vi "UHR-Fleezers Control (host) - 10.5.vi"() -> ()   [LabVIEW 2011] (continued)
          }
          frame #4 {
            n513 = property on="Trap Pos. FB ON" class="Bool (strict)"("Val(Sgnl)"=TRUE ("Value (Signaling)")) -> ()  [unwired: 2 in, 2 out]
            n514 = Wait (ms)(milliseconds to wait=u32 250) -> ()  [unwired: 1 out]
          }
          frame #5 {
            n515 = case shown="False" "Trap Trig Fl." {
              frame False {
                n516 = case shown="True" "Green ON after FB ON?" {
                  selector: "Green ON after FB ON?" -> [_ w823]
                  frame False {
                  }
                  frame True {
                    n517 = property on="Green Laser ON/Interlacing" class="Bool (strict)"("Val(Sgnl)"=w823) -> ()  [unwired: 2 in, 2 out]
                  }
                }
              }
              frame True {
              }
            }
            n518 = case shown="True" "Remove Action Offset" {
              tunnel: TRUE ("Value (Signaling)") -> [w820 w821]
              frame False {
                n519 = property on="Remove Unwinding Offset" class="Bool (strict)"("Val(Sgnl)"=w820) -> ()  [unwired: 2 in, 2 out]
              }
              frame True {
                n520 = property on="Remove Action Offset" class="Bool (strict)"("Val(Sgnl)"=w821) -> ()  [unwired: 2 in, 2 out]
              }
            }
            n521 = Wait (ms)(milliseconds to wait=u32 250) -> ()  [unwired: 1 out]
          }
          frame #6 {
            n522 = property on="Start Saving" class="Bool (strict)"("Val(Sgnl)"=TRUE ("Value (Signaling)")) -> ()  [unwired: 2 in, 2 out]
            n523 = Wait (ms)(milliseconds to wait=u32 5000) -> ()  [unwired: 1 out]
          }
          frame #7 {
            n524 = property on="Rem fb disp offset" class="Bool (strict)"("Val(Sgnl)"=TRUE ("Value (Signaling)")) -> ()  [unwired: 2 in, 2 out]
            n525 = Wait (ms)(milliseconds to wait=u32 100) -> ()  [unwired: 1 out]
          }
          frame #8 {
            n526 = case shown="True" w830 {
              frame False {
              }
              frame True {
                n527 = local write "Trap Trig. Fl."(TRUE ("Value (Signaling)")) -> ()
              }
            }
          }
          frame #9 {
            n528 = case shown="True" "Start dipping after?" {
              frame False {
              }
              frame True {
                n529 = property on="Dip for Protein" class="Bool (strict)"("Val(Sgnl)"=TRUE ("Value (Signaling)")) -> ()  [unwired: 2 in, 2 out]
                n530 = local write "Scripts"(T2."Dipping" ("Scripts")) -> ()
              }
            }
          }
        }
      }
      event "Fixed Traps Data\nScript": Value Change {
        n531 = event-data() -> ()  [unwired: 1 in, 5 out]
        n532 = flat-sequence {
          frame #0 {
            n533 = case shown="True" "Green ON" {
              frame False {
              }
              frame True {
                n534 = property on="Green Laser ON/Interlacing" class="Bool (strict)"("Val(Sgnl)"=TRUE) -> ()  [unwired: 2 in, 2 out]
              }
            }
            n535 = local write "Offset (nm)"(0.0 ("Offset (nm)")) -> ()
            n536 = property on="Sample Channel\nFlow" class="Bool (strict)"("Val(Sgnl)"=FALSE ("Value (Signaling)")) -> ()  [unwired: 2 in, 2 out]
            n537 = property on="Trap Delta (MHz)" class="DigNum (strict)"("Val(Sgnl)"="Fixed Traps Trap Delta (MHz)") -> ()  [unwired: 2 in, 2 out]
          }
          frame #1 {
            n538 = Wait (ms)(milliseconds to wait=u32 1000) -> ()  [unwired: 1 out]
          }
          frame #2 {
            n539 = local write "Start Saving"(TRUE ("Start Saving")) -> ()
          }
          frame #3 {
            n540 = local read "Bead Sep. Int. Time (s)"() -> (w842:dbl)
            n541 = Multiply(x=w842, y=1000.0) -> (x*y=w844:dbl)
            n542 = Wait (ms)(milliseconds to wait=w844) -> ()  [unwired: 1 out]
          }
          frame #4 {
            n543 = property on="Remove Offset" class="Bool (strict)"("Val(Sgnl)"=TRUE ("Value (Signaling)")) -> ()  [unwired: 2 in, 2 out]
          }
          frame #5 {
            n544 = property on="Dip for Protein" class="Bool (strict)"("Val(Sgnl)"="Start dipping after?") -> ()  [unwired: 2 in, 2 out]
          }
        }
      }
      event "Got DNA bead": Value Change {
        n545 = event-data() -> ()  [unwired: 1 in, 5 out]
        n546 = flat-sequence {
          frame #0 {
            n547 = local read "Daq spot flow on"() -> (w848:bool)
            n548 = case shown="True" w848 {
              frame False {
              }
              frame True {
                n549 = property on="Sample Channel\nFlow" class="Bool (strict)"("Val(Sgnl)"=TRUE ("Value (Signaling)")) -> ()  [unwired: 2 in, 2 out]
              }
            }
          }
          frame #1 {
            n550 = property on="Cal/Data Acq. Spot" class="Bool (strict)"("Val(Sgnl)"=TRUE ("Value (Signaling)")) -> ()  [unwired: 2 in, 2 out]
            n551 = property on="Inject Pump 1" class="Bool (strict)"("Val(Sgnl)"=FALSE ("Value (Signaling)")) -> ()  [unwired: 2 in, 2 out]
          }
        }
      }
      event "Take Stepping Data": Value Change {
        n552 = event-data() -> ()  [unwired: 1 in, 5 out]
        n553 = local read "Save ave N"() -> (w860:dbl)
        n554 = flat-sequence {
          tunnel: w860 -> [w862]
          tunnel: [w862] -> w855
          tunnel: [w864] -> w856
          tunnel: w855 -> [w864]
          tunnel: [w866] -> w857
          tunnel: w856 -> [w866]
          tunnel: [w869] -> w858
          tunnel: w857 -> [w869]
          tunnel: [w871] -> w859
          tunnel: w858 -> [w871]
          tunnel: [w873] -> w853
          tunnel: w859 -> [w873]
          tunnel: w853 -> [w876]
          tunnel: [w876] -> w852
          tunnel: w852 -> [w877]
          tunnel: [w877] -> w854
          tunnel: w854 -> [w883]
          frame #0 {
            n555 = property on="Save ave N" class="DigNum (strict)"("Val(Sgnl)"="Save ave factor") -> ()  [unwired: 2 in, 2 out]
          }
          frame #1 {
            n556 = Wait (ms)(milliseconds to wait=u32 100) -> ()  [unwired: 1 out]
          }
          frame #2 {
            n557 = local read "Offset 2 Start (MHz)"() -> (w868:dbl)
            n558 = property on="Saved AOD Raster Scan Parameter Sets" class="Arr (strict)"("Index Values"=u32[] [2]) -> ()  [unwired: 2 in, 2 out]
            n559 = property on="Trap Delta (MHz)" class="DigNum (strict)"("Val(Sgnl)"=w868) -> ()  [unwired: 2 in, 2 out]
          }
          frame #3 {
            n560 = property on="Load parameters" class="Bool (strict)"("Val(Sgnl)"=TRUE ("Value (Signaling)")) -> ()  [unwired: 2 in, 2 out]
          }
          frame #4 {
            n561 = Wait (ms)(milliseconds to wait=u32 100) -> ()  [unwired: 1 out]
          }
          frame #5 {
            n562 = property on="Trap Raster Scan" class="Bool (strict)"("Val(Sgnl)"=TRUE ("Value (Signaling)")) -> ()  [unwired: 2 in, 2 out]
          }
          frame #6 {
            n563 = Wait (ms)(milliseconds to wait=u32 1000) -> ()  [unwired: 1 out]
          }
          frame #7 {
            n564 = while {
              stop <- w880 stop-if-true
              n565 = local read "Raster Scanning..."() -> (w882:bool)
              n566 = local read "Saving..."() -> (w881:bool)
              n567 = Not(x=w881) -> (.not. x?=w878:bool)
              n568 = Not(x=w882) -> (.not. x?=w879:bool)
              n569 = And(x=w879, y=w878) -> (x .and. y?=w880:bool)
            }
          }
          frame #8 {
            n570 = property on="Save ave N" class="DigNum (strict)"("Val(Sgnl)"=w883) -> ()  [unwired: 2 in, 2 out]
          }
        }
      }
      event "Step Size (nm)": Value Change {
        n571 = event-data() -> ()  [unwired: 1 in, 5 out]
        n572 = flat-sequence {
          frame #0 {
            n573 = property on="Saved AOD Raster Scan Parameter Sets" class="Arr (strict)"("Index Values"=u32[] [1]) -> ()  [unwired: 2 in, 2 out]
          }
          frame #1 {
            n574 = Multiply(x="N Steps", y="Step Size (nm)") -> (x*y=w885:dbl)
            n575 = property on="Scan Speed AOD (nm/s) 2" class="DigNum (strict)"("Value"="Step Size (nm)") -> ()  [unwired: 2 in, 2 out]
            n576 = property on="Step Size AOD (nm) 2" class="DigNum (strict)"("Value"="Step Size (nm)") -> ()  [unwired: 2 in, 2 out]
            n577 = property on="Scan Range AOD (nm) 2" class="DigNum (strict)"("Value"=w885) -> ()  [unwired: 2 in, 2 out]
          }
        }
      }
      event "Take Detection Laser\nImage": Value Change {
        n578 = event-data() -> ()  [unwired: 1 in, 5 out]
        n579 = flat-sequence {
          tunnel: [w913] -> w903
          tunnel: [w912] -> w896
          tunnel: [w911] -> w888
          tunnel: [w916] -> w904
          tunnel: w903 -> [w916]
          tunnel: [w915] -> w897
          tunnel: w896 -> [w915]
          tunnel: [w914] -> w889
          tunnel: w888 -> [w914]
          tunnel: [w920] -> w905
          tunnel: w904 -> [w920]
          tunnel: [w919] -> w898
          tunnel: w897 -> [w919]
          tunnel: [w918] -> w890
          tunnel: w889 -> [w918]
          tunnel: [w926] -> w906
          tunnel: w905 -> [w926]
          tunnel: [w925] -> w899
          tunnel: w898 -> [w925]
          tunnel: [w924] -> w891
          tunnel: w890 -> [w924]
          tunnel: [w930] -> w907
          tunnel: w906 -> [w930]
          tunnel: [w929] -> w900
          tunnel: w899 -> [w929]
          tunnel: [w928] -> w892
          tunnel: w891 -> [w928]
          tunnel: [w934] -> w908
          tunnel: w907 -> [w934]
          tunnel: [w933] -> w901
          tunnel: w900 -> [w933]
          tunnel: [w932] -> w893
          tunnel: w892 -> [w932]
          tunnel: [w938] -> w909
          tunnel: w908 -> [w938]
          tunnel: [w937] -> w902
          tunnel: w901 -> [w937]
          tunnel: [w936] -> w894
          tunnel: w893 -> [w936]
          tunnel: w909 -> [w944]
          tunnel: w902 -> [w943]
          tunnel: [w941] -> w895
          tunnel: w894 -> [w941]
          tunnel: w895 -> [w945]
          frame #0 {
            n580 = local read "Green Laser ON/Interlacing"() -> (w913:bool)
            n581 = local read "Green laser mode"() -> (w912:enum32{"Laser ON", "Laser OFF", "Interlace"})
            n582 = local read "Green FB On/Off"() -> (w911:bool)
          }
          frame #1 {
            n583 = property on="Green FB On/Off" class="Bool (strict)"("Val(Sgnl)"=FALSE ("Value (Signaling)")) -> ()  [unwired: 2 in, 2 out]
          }
          frame #2 {
            n584 = property on="Green Laser ON/Interlacing" class="Bool (strict)"("Val(Sgnl)"=TRUE ("Value (Signaling)")) -> ()  [unwired: 2 in, 2 out]
            n585 = property on="Flip Green Filter" class="Bool (strict)"("Val(Sgnl)"=TRUE ("Value (Signaling)")) -> ()  [unwired: 2 in, 2 out]
            n586 = property on="Green laser mode" class="RadioBtnsControl (strict)"("Val(Sgnl)"=enum32{"Laser ON", "Laser OFF", "Interlace"}."Laser ON" ("Value (Signaling)")) -> ()  [unwired: 2 in, 2 out]
          }
          frame #3 {
            n587 = Wait (ms)(milliseconds to wait=u32 500) -> ()  [unwired: 1 out]
          }
          frame #4 {
            n588 = property on="Confocal Image" class="Bool (strict)"("Val(Sgnl)"=TRUE ("Value (Signaling)")) -> ()  [unwired: 2 in, 2 out]
          }
          frame #5 {
            n589 = Wait (ms)(milliseconds to wait=u32 2000) -> ()  [unwired: 1 out]
          }
          frame #6 {
            n590 = while {
              stop <- w939 stop-if-true
              n591 = local read "Saving..."() -> (w940:bool)
              n592 = Not(x=w940) -> (.not. x?=w939:bool)
            }
          }
          frame #7 {
            n593 = property on="Flip Green Filter" class="Bool (strict)"("Val(Sgnl)"=TRUE ("Value (Signaling)")) -> ()  [unwired: 2 in, 2 out]
            n594 = property on="Green Laser ON/Interlacing" class="Bool (strict)"("Val(Sgnl)"=w944) -> ()  [unwired: 2 in, 2 out]
            n595 = property on="Green laser mode" class="RadioBtnsControl (strict)"("Val(Sgnl)"=w943) -> ()  [unwired: 2 in, 2 out]
          }
          frame #8 {
            n596 = property on="Green FB On/Off" class="Bool (strict)"("Val(Sgnl)"=w945) -> ()  [unwired: 2 in, 2 out]
          }
        }
      }
      event "Stop All": Value Change {
        n597 = event-data() -> ()  [unwired: 1 in, 5 out]
        n598 = local read "Stop All"() -> (w946:bool)
      }
    }
    n599 = node-c288() -> ()  [unwired: 1 in, 1 out]
  }
  n600 = node-c288(2 ("Processor")) -> (w82:T21)  [unwired: 3 out]
  n601 = timed-loop "Control parameters (event loop)" {
    tunnel: w40 -> [w951]
    shift-right: [w950] -> _
    shift-left: errorcluster {"status"=FALSE, "code"=0, "source"=""} ("error out") -> [w949]
    tunnel: [w948] -> _
    timing: w82 -> [_]
    timing-out: [_] -> w81
    tunnel: w54 -> [w947]
    stop <- w948 stop-if-true
    n602 = node-c288() -> ()  [unwired: 2 out]
    n603 = event shown="[44] \"Sample Channel\nFlow\": Value Change" {
      selector: _ -> [_ _ _ _ _ _ _ _ _ _ _ _ _ _ _ _ _ _ _ _ _ _ _ _ _ _ _ _ _ _ _ _ _ _ _ _ _ _ _ _ _ _ _ _ _ _ _ _ _ _ _ _ _ _ _ _ _ _ _ _ _ _ _]
      dyn-events: _ -> [_ _ _ _ _ _ _ _ _ _ _ _ _ _ _ _ _ _ _ _ _ _ _ _ _ _ _ _ _ _ _ _ _ _ _ _ _ _ _ _ _ _ _ _ _ _ _ _ _ _ _ _ _ _ _ _ _ _ _ _ _ _ _]
      timeout: _ -> [_ _ _ _ _ _ _ _ _ _ _ _ _ _ _ _ _ _ _ _ _ _ _ _ _ _ _ _ _ _ _ _ _ _ _ _ _ _ _ _ _ _ _ _ _ _ _ _ _ _ _ _ _ _ _ _ _ _ _ _ _ _ _]
      tunnel: w951 -> [w989 _ _ _ w1027 _ w1049 _ _ _ _ w1115 _ _ w1158 w1164 w1169 w1175 w1211 w1229 w1236 w1247 w1251 w1262 w1273 w1284 w1295 w1306 w1317 w1344 w1438 w1445 w1483 _ w1518 w1522 w1533 w1537 w1541 _ w1549 _ _ _ _ _ _ _ w1720 _ w1737 _ w1744 w1762 _ w1769 w1777 w1792 w1803 w1806 w1811 _ w1830]
      tunnel: [w988 _ _ _ w1017 _ w1048 _ _ w1080 _ w1094 _ _ w1157 w1160 w1166 w1172 w1210 w1227 w1235 w1245 _ w1256 w1267 w1278 w1289 w1300 w1311 w1342 w1436 w1443 w1481 _ w1516 w1520 w1523 w1535 w1539 _ w1547 _ _ _ _ _ _ _ w1718 _ _ _ _ w1759 _ _ _ _ _ _ _ _ _] -> w950
      tunnel: w949 -> [w987 _ _ _ w1026 _ w1047 _ _ w1080 _ w1114 _ _ w1156 w1159 w1165 w1171 w1209 w1228 w1234 w1246 w1250 w1261 w1272 w1283 w1294 w1305 w1316 w1343 w1437 w1444 w1482 _ w1517 w1521 w1532 w1536 w1540 _ w1548 _ _ _ _ _ _ _ w1719 _ w1736 _ w1743 w1761 _ w1768 w1776 w1791 w1802 w1805 w1810 _ w1829]
      tunnel: [_ _ _ _ _ _ _ _ _ w1079 _ _ _ _ _ _ _ _ _ _ _ _ _ _ _ _ _ _ _ _ _ _ _ _ _ _ _ _ _ _ _ _ _ _ _ _ _ _ _ _ _ _ _ _ _ _ _ _ _ _ _ _ _] -> w948
      tunnel: [_ _ _ _ _ _ _ "Round T1 X" _ _ _ _ _ _ _ _ _ _ _ _ _ _ _ _ _ _ _ _ _ _ _ _ _ _ _ _ _ _ _ _ _ _ _ _ _ _ _ _ _ _ _ _ _ _ _ _ _ _ _ _ _ _ _] -> _
      tunnel: [_ _ _ "Adjust Scale\nto Mean" _ _ _ _ _ _ _ _ _ _ _ _ _ _ _ _ _ "Test ttrig" _ _ _ _ _ _ _ _ _ _ _ _ _ _ _ _ _ _ _ _ _ _ _ _ "Flush Sample" "Clear Volume" _ _ _ _ _ _ _ _ _ _ _ _ _ _ _] -> _
      tunnel: [_ _ _ _ _ _ _ _ "Round T2 X" _ "Delayed Interlace Start" _ _ _ _ _ _ _ _ _ _ _ _ _ _ _ _ _ _ _ _ _ _ _ _ _ _ _ _ _ _ _ _ _ _ _ _ _ _ _ _ _ _ _ _ _ _ _ _ _ _ _ _] -> _
      tunnel: w947 -> [_ _ _ _ _ _ _ _ _ _ _ _ _ _ _ _ _ _ _ _ _ _ _ _ _ _ _ _ _ _ _ _ _ _ _ _ _ _ _ _ _ _ _ _ w1662 w1677 w1705 w1707 _ _ _ _ _ _ _ _ _ _ _ _ _ _ _]
      event "AI Count (ticks)", "Sets to FIFO (Traps)", "Save ave N", "FPGA Ave.", "# Samples/channel", "N sets to save": Value Change {
        # "So that if 'Save ave N' is updated, the AOD scanning code updates too."
        n604 = event-data() -> ()  [unwired: 6 out]
        n605 = local read "AI Count (ticks)"() -> (w969:u32)
        n606 = Boolean To (0,1)(Boolean="Sets to FIFO (Traps)") -> (0, 1=w979:cluster{"Set 1":i16, "Set 2":i16, "Set 3":i16})
        n607 = xnode "Read/Write Control"("FPGA VI Reference In"=w989, "error in"=w987, "ai count"=w969, "AI1 Sets to FIFO"="Sets to FIFO (Traps)", "N of AI1 Int Acq Sets"="N Acq Sets (Traps + Fl.)") -> ("error out"=w988:errorcluster)  [unwired: 1 out]
        n608 = Cluster To Array(cluster=w979) -> (array=w978:i16[])
        n609 = To Unsigned Long Integer(number=w978) -> (unsigned 32bit integer=w958:u32[])
        n610 = local read "Scan steps (AOD)"() -> (w980:u64)
        n611 = Multiply(x=w969, y="N Acq Sets (Traps + Fl.)") -> (x*y=w967:u32)
        n612 = Divide(x=40000000.0, y=w969) -> (x/y=w961:dbl)
        "AI rate (Hz)" <- w961
        "Ave. Rate (Hz)" <- w961
        n613 = Add Array Elements(numeric array=w958) -> (sum=w970:u32)
        "Trap Sets" <- w970
        n614 = Reciprocal(x=w961) -> (1/x=→"Ave. Period (s)":dbl)
        n615 = property on="Scan steps (AOD)" class="DigNum (strict)"("Val(Sgnl)"=w980) -> ()  [unwired: 2 in, 2 out]
        n616 = Divide(x=w961, y="N Acq Sets (Traps + Fl.)") -> (x/y=w984:dbl)
        "Data Rate (Hz)" <- w984
        n617 = Reciprocal(x=w984) -> (1/x=→"Data Period (s)":dbl)
        n618 = local read "Save ave N"() -> (w983:dbl)
        n619 = Divide(x=w984, y=w983) -> (x/y=w982:dbl)
        "Save Data Rate (Hz)" <- w982
        n620 = Reciprocal(x=w982) -> (1/x=→"Save Data Period (s)":dbl)
        n621 = Multiply(x=w967, y="# Samples/trap") -> (x*y=w965:u32)
        "Counts/DMA" <- w965
        n622 = property on="Trap Disp. Downsample" class="DigNum (strict)"("Maximum"="# Samples/trap") -> ()  [unwired: 2 in, 2 out]
        n623 = Multiply(x=w970, y="# Samples/trap") -> (x*y=w959:u32)
        "# Samples/channel" <- w959
        n624 = Multiply(x=w959, y=u32 8) -> (x*y=→"Trap AI Elements/DMA read":u32)
        n625 = local read "APD Int. Count"() -> (w966:u32)
        n626 = Multiply(x=w959, y=u32 3) -> (x*y=→"Trap Pos Elements/DMA read":u32)
        n627 = Divide(x=w965, y=w966) -> (x/y=w956:dbl)
        "APD Samples/FIFO Acq." <- w956
        n628 = Divide(x=w965, y=40000000.0) -> (x/y=w963:dbl)
        "DMA Update Period (s)" <- w963
        n629 = Multiply(x=2.0, y=w956) -> (x*y=→"APD Elements/DMA read":dbl)
        n630 = property on="APD Disp. Downsample" class="DigNum (strict)"("Maximum"=w956) -> ()  [unwired: 2 in, 2 out]
        n631 = local read "N sets to save"() -> (w976:u32)
        n632 = Multiply(x=w963, y=w976) -> (x*y=→"Total Time (s)":dbl)
        "FPGA Averaging" <- FALSE ("FPGA Averaging")
      }
      event "Remove Offset": Value Change {
        n633 = event-data() -> ()  [unwired: 7 out]
        n634 = local write "Remove Offset"(FALSE ("Remove Offset")) -> ()
        n635 = local read "Bead Mean (nm)"() -> (w991:dbl)
        n636 = local read "Offset (nm)"() -> (w992:dbl)
        n637 = Add(x=w991, y=w992) -> (x+y=w990:dbl)
        n638 = local write "Offset (nm)"(w990) -> ()
        n639 = disable-structure shown="Disabled" {
          frame Disabled {
            n640 = local read "Bead Mean (nm)"() -> (w997:dbl)
            n641 = Add(y=w997) -> (x=w996:dbl, x+y=w995:dbl)
            n642 = Subtract(x=w997, y=w996) -> (x-y=w994:dbl)
            n643 = property on="Bead Separation" class="WFChart (strict)"("YScale.Minimum"=w994) -> ()  [unwired: 2 in, 2 out]
            n644 = property on="Bead Separation" class="WFChart (strict)"("YScale.Maximum"=w995) -> ()  [unwired: 2 in, 2 out]
          }
          frame Enabled {
          }
        }
      }
      event "Detector Type": Value Change {
        n645 = event-data() -> ()  [unwired: 7 out]
        n646 = local read "AI labels"() -> (w998:string[])
        n647 = property on="High Res. Display" class="Ring (strict)"("Strings []"=w998) -> ()  [unwired: 2 in, 2 out]
        n648 = Build Array (concatenate)(w998, "none") -> (w999:string[])
        n649 = property on="FFT 1 Choice 1" class="Ring (strict)"("Strings []"=w999) -> ()  [unwired: 2 in, 2 out]
        n650 = property on="FFT 1 Choice 2" class="Ring (strict)"("Strings []"=w999) -> ()  [unwired: 2 in, 2 out]
        n651 = property on="FFT 2 Choice 1" class="Ring (strict)"("Strings []"=w999) -> ()  [unwired: 2 in, 2 out]
        n652 = property on="FFT 2 Choice 2" class="Ring (strict)"("Strings []"=w999) -> ()  [unwired: 2 in, 2 out]
        n653 = Bundle("APD 1", "APD 2") -> (w1002:cluster{string, string})  [unwired: 1 out]
        n654 = Cluster To Array(cluster=w1002) -> (array=w1000:string[])
        n655 = Build Array (concatenate)(w1000, w999) -> (w1004:string[])
        n656 = Array Size(array=w1004) -> (size(s)=w1005:i32)
        n657 = property on="Signals to Plot" class="LstBox (strict)"("Item Names"=w1004) -> ()  [unwired: 2 in, 2 out]
        n658 = property on="Signals to Plot" class="LstBox (strict)"("Number of Rows"=w1005) -> ()  [unwired: 2 in, 2 out]
        n659 = property on="All Signals" class="WFChart (strict)"("LegNumRows"=w1005) -> ()  [unwired: 2 in, 2 out]
      }
      event "Adjust Scale\nto Mean": Value Change {
        n660 = event-data() -> ()  [unwired: 7 out]
        n661 = local read "APD 1 Rate (Hz)"() -> (w1014:dbl)
        n662 = Multiply(x=1000.0, y="Above (kHz)") -> (x*y=w1012:dbl)
        n663 = Multiply(x=1000.0, y="Below (kHz)") -> (x*y=w1010:dbl)
        n664 = Add(x=w1012, y=w1014) -> (x+y=w1007:dbl)
        n665 = Subtract(x=w1014, y=w1010) -> (x-y=w1008:dbl)
        n666 = property on="APD Chart" class="WFChart (strict)"("YScale.Minimum"=w1008) -> ()  [unwired: 2 in, 2 out]
        n667 = property on="APD Chart" class="WFChart (strict)"("YScale.Maximum"=w1007) -> ()  [unwired: 2 in, 2 out]
      }
      event "Phase adj. (AI1)", "+ phase (AI1)", "- phase (AI1)": Value Change {
        n668 = event-data() -> ()  [unwired: 7 out]
        n669 = Negate(x="Phase adj. (AI1)") -> (-x=w1024:i16)
        n670 = Select(t=w1024, s="- phase (AI1)", f="Phase adj. (AI1)") -> (s? t:f=w1023:i16)
        n671 = xnode "Read/Write Control"("FPGA VI Reference In"=w1027, "error in"=w1026, "Phase count adjustment"=w1023) -> ("FPGA VI Reference Out"=w1022:T19, "error out"=w1021:errorcluster)
        n672 = Or(x="- phase (AI1)", y="+ phase (AI1)") -> (x .or. y?=w1018:bool)
        n673 = xnode "Read/Write Control"("FPGA VI Reference In"=w1022, "error in"=w1021, "+ phase"=w1018) -> ("error out"=w1017:errorcluster)  [unwired: 1 out]
      }
      event "Signals to Plot": Double Click {
        w1030 = u32 9868950 ("Color Box")
        n674 = event-data() -> ("Row"=w1032:i32)  [unwired: 9 out]
        n675 = property on="All Signals" class="WFChart (strict)"("Active Plot"=w1032) -> (error out=w1043:errorcluster)  [unwired: 2 in, 1 out]
        n676 = property on="All Signals" class="WFChart (strict)" props=["Plot", "Visible?", "Plot", "Plot Color"](error in=w1043) -> (error out=w1042:errorcluster, "Plot.Visible?"=w1041:bool)  [unwired: 1 in, 2 out]
        n677 = Select(t=FALSE ("Plot.Visible"), s=w1041, f=TRUE ("Plot.Visible")) -> (s? t:f=w1036:bool)
        n678 = property on="All Signals" class="WFChart (strict)"(error in=w1042, "Plot.Visible?"=w1036) -> (error out=w1038:errorcluster)  [unwired: 1 in, 1 out]
        n679 = property on="All Signals" class="WFChart (strict)"(error in=w1038) -> (error out=w1033:errorcluster, "Plot.Plot Color"=w1037:u32)  [unwired: 1 in, 1 out]
        n680 = property on="Signals to Plot" class="LstBox (strict)"(error in=w1033, "Active Row"=w1032) -> (error out=w1031:errorcluster)  [unwired: 1 in, 1 out]
        n681 = Select(t=w1037, s=w1036, f=u32 0) -> (s? t:f=w1034:u32)
        n682 = property on="Signals to Plot" class="LstBox (strict)"(error in=w1031, "CellFontColor"=w1034, "SelColor"=w1030, "CellBG"=w1030, "CellFontSize"=u32 20 ("Active Row:Cell Font:Size"), "CellFontBold"=TRUE ("Active Row:Cell Font:Bold")) -> ()  [unwired: 1 in, 2 out]
      }
      event "BD 1 Frequency 1 (MHz)", "BD 1 Frequency 2 (MHz)", "BD 1 Frequency 3 (MHz)", "BD 2 Frequency 1 (MHz)", "BD 2 Frequency 2 (MHz)", "BD 2 Frequency 3 (MHz)", "Trap Delta (MHz)": Value Change {
        n683 = event-data() -> ("CtlRef"=w1046:refnum<vi>)  [unwired: 6 out]
        n684 = control-ref of="Trap Delta (MHz)"() -> (w1045:refnum<vi>)
        n685 = Equal?(x=w1045, y=w1046) -> (x = y?=w1044:bool)
        n686 = case shown="False" "Oscillate Set 1" {
          tunnel: w1049 -> [w1069 _]
          tunnel: [w1068 w1072] -> w1048
          tunnel: w1047 -> [w1067 w1072]
          tunnel: w1044 -> [w1052 _]
          frame False {
            n687 = local read "BD 1 Frequency 2 (MHz)"() -> (w1056:dbl)
            n688 = local read "BD 1 Frequency 1 (MHz)"() -> (w1054:dbl)
            n689 = Subtract(x=w1056, y="Trap Delta (MHz)") -> (x-y=w1053:dbl)
            n690 = Select(t=w1053, s=w1052, f=w1054) -> (s? t:f=w1051:dbl)
            n691 = local read "Y RF Frequency Limits (MHz)"() -> (w1057:T16)
            n692 = local read "X RF Frequency Limits (MHz)"() -> (w1058:T16)
            n693 = local read "BD 1 Frequency 3 (MHz)"() -> (w1070:dbl)
            n694 = local write "BD 1 Frequency 1 (MHz)"(w1051) -> ()
            n695 = local read "BD 2 Frequency 1 (MHz)"() -> (w1061:dbl)
            n696 = local read "BD 2 Frequency 2 (MHz)"() -> (w1060:dbl)
            n697 = local read "BD 2 Frequency 3 (MHz)"() -> (w1071:dbl)
            n698 = call "set RF board frequency - interlace.vi"("Board 2 Frequency Limits"=w1057, "Board 1 Frequency Limits"=w1058, "error in"=w1067, "FPGA VI Reference In"=w1069, "Board 2 Frequency 3 (MHz)"=w1071, "Board 1 Frequency 3 (MHz)"=w1070, "Board 2 Frequency 2 (MHz)"=w1060, "Board 2 Frequency 1 (MHz)"=w1061, "Board 1 Frequency 2 (MHz)"=w1056, "Board 1 Frequency 1  (MHz)"=w1051) -> ("error out"=w1068:errorcluster)  [unwired: 1 out]
            n699 = Subtract(x=w1061, y=w1060) -> (x-y=w1065:dbl)
            n700 = Subtract(x=w1051, y=w1056) -> (x-y=w1066:dbl)
            n701 = Square(x=w1065) -> (x^2=w1063:dbl)
            n702 = Square(x=w1066) -> (x^2=w1064:dbl)
            n703 = Add(x=w1064, y=w1063) -> (x+y=w1062:dbl)
            n704 = Square Root(x=w1062) -> (sqrt(x)=w1059:dbl)
            n705 = local write "Trap Delta (MHz)"(w1059) -> ()
            n706 = property on="Initial delta (MHz)" class="DigNum (strict)"("Val(Sgnl)"=w1059) -> ()  [unwired: 2 in, 2 out]
          }
          frame True {
          }
        }
      }
      event "Round T1 X": Value Change {
        n707 = event-data() -> ()  [unwired: 7 out]
        n708 = local read "BD 1 Frequency 1 (MHz)"() -> (w1075:dbl)
        n709 = Round To Nearest(number=w1075) -> (nearest integer value=w1074:dbl)
        n710 = property on="BD 1 Frequency 1 (MHz)" class="DigNum (strict)"("Val(Sgnl)"=w1074) -> ()  [unwired: 2 in, 2 out]
      }
      event "Round T2 X": Value Change {
        n711 = event-data() -> ()  [unwired: 7 out]
        n712 = local read "BD 1 Frequency 2 (MHz)"() -> (w1077:dbl)
        n713 = Round To Nearest(number=w1077) -> (nearest integer value=w1076:dbl)
        n714 = property on="BD 1 Frequency 2 (MHz)" class="DigNum (strict)"("Val(Sgnl)"=w1076) -> ()  [unwired: 2 in, 2 out]
      }
      event "Stop All": Value Change {
        n715 = event-data() -> ()  [unwired: 7 out]
        n716 = local read "Stop All"() -> (w1079:bool)
      }
      event "Delayed Interlace Start": Value Change {
        n717 = event-data() -> ()  [unwired: 7 out]
        n718 = flat-sequence {
          frame #0 {
            n719 = Multiply(x="Delay to Interlace (s)", y=1000.0) -> (x*y=w1082:dbl)
            n720 = Wait (ms)(milliseconds to wait=w1082) -> ()  [unwired: 1 out]
          }
          frame #1 {
            n721 = property on="Green laser mode" class="RadioBtnsControl (strict)"("Val(Sgnl)"=enum32{"Laser ON", "Laser OFF", "Interlace"}."Interlace" ("Value (Signaling)")) -> ()  [unwired: 2 in, 2 out]
          }
        }
      }
      event "BD 1 Amplitude 1 (%)", "BD 1 Amplitude 2 (%)", "BD 1 Amplitude 3 (%)", "BD 2 Amplitude 1 (%)", "BD 2 Amplitude 2 (%)", "BD 2 Amplitude 3 (%)", "Trap 1 ON", "Trap 2 ON", "Trap 3 ON", "Feedback On/Off", "All FB On/Off": Value Change {
        w1106 = i16 1 ("f")
        n722 = event-data() -> ()  [unwired: 7 out]
        n723 = local write "Trap 1 (ON/OFF)"("Trap 1 ON") -> ()
        n724 = local write "Trap 2 (ON/OFF)"("Trap 2 ON") -> ()
        n725 = Boolean To (0,1)(Boolean="Trap 3 ON") -> (0, 1=w1107:i16)
        n726 = Boolean To (0,1)(Boolean="Trap 1 ON") -> (0, 1=w1108:i16)
        n727 = Boolean To (0,1)(Boolean="Trap 2 ON") -> (0, 1=w1109:i16)
        n728 = Select(t=w1109, s="Trap ON/OFF X or Y Amp?", f=w1106) -> (s? t:f=w1104:i16)
        n729 = Select(t=w1108, s="Trap ON/OFF X or Y Amp?", f=w1106) -> (s? t:f=w1105:i16)
        n730 = Select(t=w1107, s="Trap ON/OFF X or Y Amp?", f=w1106) -> (s? t:f=w1103:i16)
        n731 = Select(t=w1106, s="Trap ON/OFF X or Y Amp?", f=w1109) -> (s? t:f=w1101:i16)
        n732 = Select(t=w1106, s="Trap ON/OFF X or Y Amp?", f=w1108) -> (s? t:f=w1102:i16)
        n733 = Select(t=w1106, s="Trap ON/OFF X or Y Amp?", f=w1107) -> (s? t:f=w1100:i16)
        n734 = And(x="All FB On/Off", y="Feedback On/Off") -> (x .and. y?=w1098:cluster{"Set 1":bool, "Set 2":bool})
        n735 = local read "BD 1 Amplitude 1 (%)"() -> (w1118:dbl)
        n736 = local read "BD 1 Amplitude 2 (%)"() -> (w1117:dbl)
        n737 = local read "BD 1 Amplitude 3 (%)"() -> (w1116:dbl)
        n738 = Unbundle By Name(w1098) -> ("Set 1"=w1093:bool, "Set 2"=w1090:bool)
        n739 = local read "Y RF Amplitude Limits (%)"() -> (w1086:T16)
        n740 = local read "X RF Amplitude Limits (%)"() -> (w1087:T16)
        n741 = local read "BD 2 Amplitude 1 (%)"() -> (w1119:dbl)
        n742 = local read "BD 2 Amplitude 2 (%)"() -> (w1120:dbl)
        n743 = local read "BD 2 Amplitude 3 (%)"() -> (w1121:dbl)
        n744 = And(x="Trap 2 ON", y=w1090) -> (x .and. y?=w1088:bool)
        n745 = And(x="Trap 1 ON", y=w1093) -> (x .and. y?=w1091:bool)
        n746 = Multiply(x=w1105, y=w1118) -> (x*y=w1113:dbl)
        n747 = Multiply(x=w1117, y=w1104) -> (x*y=w1111:dbl)
        n748 = Multiply(x=w1116, y=w1103) -> (x*y=w1112:dbl)
        n749 = Multiply(x=w1119, y=w1102) -> (x*y=w1122:dbl)
        n750 = Multiply(x=w1120, y=w1101) -> (x*y=w1123:dbl)
        n751 = Multiply(x=w1121, y=w1100) -> (x*y=w1124:dbl)
        n752 = call "set RF board amplitude - interlace.vi"("Board 2 Amplitude Limits"=w1086, "Board 1 Amplitude Limits"=w1087, "error in"=w1114, "FPGA VI Reference In"=w1115, "Board 2 Amplitude 3 (%)"=w1124, "Board 1 Amplitude 3 (%)"=w1112, "Board 2 Amplitude 2 (%)"=w1123, "Board 2 Amplitude 1 (%)"=w1122, "Board 1 Amplitude 2 (%)"=w1111, "Board 1 Amplitude 1 (%)"=w1113) -> ("error out"=w1095:errorcluster, "FPGA VI Reference Out"=w1096:T19)
        n753 = xnode "Read/Write Control"("FPGA VI Reference In"=w1096, "error in"=w1095, "FB On/Off Set 1"=w1091, "FB On/Off Set 2"=w1088) -> ("error out"=w1094:errorcluster)  [unwired: 1 out]
      }
      event "Load parameters": Value Change {
        n754 = event-data() -> ()  [unwired: 7 out]
        n755 = property on="Saved AOD Raster Scan Parameter Sets" class="Arr (strict)"() -> ("Index Values"=w1135:u32[])  [unwired: 2 in, 2 out]
        n756 = Index Array(array=w1135, index=0) -> (element=w1132:u32)
        n757 = local write "Load parameters"(FALSE ("Load parameters")) -> ()
        n758 = Index Array(array="Saved AOD Raster Scan Parameter Sets", index=w1132) -> (element=w1131:T26)
        n759 = Unbundle By Name(w1131) -> ("Scan Range AOD (nm) 2"=w1130:dbl, "Step Size AOD (nm) 2"=w1129:dbl, "Scan Speed AOD (nm/s) 2"=w1128:dbl, "Number of scans (AOD) 2"=w1127:u16)
        n760 = flat-sequence {
          tunnel: w1130 -> [w1138]
          tunnel: w1129 -> [w1137]
          tunnel: w1128 -> [w1136]
          tunnel: w1127 -> [w1139]
          frame #0 {
            n761 = local write "Scan Speed (nm/s)"(w1136) -> ()
            n762 = local write "Scan Range (nm)"(w1138) -> ()
            n763 = local write "Step Size (nm)"(w1137) -> ()
          }
          frame #1 {
            n764 = property on="Number of F/B Scans (AOD)" class="DigNum (strict)"("Val(Sgnl)"=w1139) -> ()  [unwired: 2 in, 2 out]
          }
        }
      }
      event "Trap 1 (ON/OFF)", "Trap 2 (ON/OFF)": Value Change {
        n765 = event-data() -> ()  [unwired: 7 out]
        n766 = property on="Trap 2 ON" class="Bool (strict)"("Val(Sgnl)"="Trap 2 (ON/OFF)") -> ()  [unwired: 2 in, 2 out]
        n767 = property on="Trap 1 ON" class="Bool (strict)"("Val(Sgnl)"="Trap 1 (ON/OFF)") -> ()  [unwired: 2 in, 2 out]
      }
      event "DIO count 1 (ticks)", "DIO count 2 (ticks)", "DIO count 3 (ticks)", "Interlace", "Number Interlace Sets", "Not-Interlacing Set": Value Change {
        n768 = event-data() -> ()  [unwired: 7 out]
        n769 = local read "DIO count 3 (ticks)"() -> (w1152:u32)
        n770 = local read "DIO count 1 (ticks)"() -> (w1154:u32)
        n771 = local read "DIO count 2 (ticks)"() -> (w1153:u32)
        n772 = To Unsigned Byte Integer(number="Not-Interlacing Set") -> (unsigned 8bit integer=w1143:u8)
        n773 = Add(x=w1143, y=u8 1) -> (x+y=w1147:u8)
        n774 = xnode "Read/Write Control"("FPGA VI Reference In"=w1158, "error in"=w1156, "DIO count 1 (ticks)"=w1154, "DIO count 2 (ticks)"=w1153, "DIO count 3 (ticks)"=w1152, "Interlace ON/OFF"="Interlace", "Number Interlace Cycles"="Number Interlace Sets", "Interlace Off Parameters"=w1147) -> ("error out"=w1157:errorcluster)  [unwired: 1 out]
        n775 = Build Array(w1154, w1153, w1152) -> (w1145:u32[])
        n776 = Split 1D Array(array=w1145, index="Number Interlace Sets") -> (first subarray=w1155:u32[])  [unwired: 1 out]
        n777 = Index Array(array=w1145, index=w1143) -> (element=w1144:u32)
        n778 = Add Array Elements(numeric array=w1155) -> (sum=w1149:u32)
        n779 = Select(t=w1149, s="Interlace", f=w1144) -> (s? t:f=→"Total Counts (ticks)":u32)
      }
      event "Reset Feedback": Value Change {
        n780 = event-data() -> ()  [unwired: 7 out]
        n781 = Unbundle By Name("Reset Feedback") -> ("Set 1"=w1162:bool, "Set 2"=w1161:bool)
        n782 = xnode "Read/Write Control"("FPGA VI Reference In"=w1164, "error in"=w1159, "FB Reset Set 1"=w1162, "FB Reset Set 2"=w1161) -> ("error out"=w1160:errorcluster)  [unwired: 1 out]
      }
      event "PID Gains": Value Change {
        n783 = event-data() -> ()  [unwired: 7 out]
        n784 = Unbundle By Name("PID Gains") -> ("Set 1"=w1168:T14, "Set 2"=w1167:T14)
        n785 = xnode "Read/Write Control"("FPGA VI Reference In"=w1169, "error in"=w1165, "FB Gains Set 1"=w1168, "FB Gains Set 2"=w1167) -> ("error out"=w1166:errorcluster)  [unwired: 1 out]
      }
      event "AI2 to Setpoint", "Setpoints (V)": Value Change {
        n786 = event-data() -> ()  [unwired: 7 out]
        n787 = xnode "Read/Write Control"("FPGA VI Reference In"=w1175, "error in"=w1171) -> ("FPGA VI Reference Out"=w1174:T19, "error out"=w1173:errorcluster, "AI2 Y Sum Set 1"=w1182:i16, "AI2 Y Sum Set 2"=w1181:i16)
        n788 = Cluster To Array(cluster="AI2 to Setpoint") -> (array=w1185:bool[])
        n789 = local read "AI2 (V)"() -> (w1183:cluster{"Set 1":dbl, "Set 2":dbl})
        n790 = Or Array Elements(Boolean array=w1185) -> (logical OR=w1186:bool)
        n791 = Bundle By Name(cluster=w1183, "Set 1"=w1182, "Set 2"=w1181) -> (w1180:cluster{"Set 1":dbl, "Set 2":dbl})
        n792 = Divide(x=w1180, y=3276.7) -> (x/y=w1179:cluster{"Set 1":dbl, "Set 2":dbl})
        "AI2 (V)" <- w1179
        n793 = case shown="True" w1186 {
          tunnel: [w1189 w1206] -> w1178
          tunnel: "AI2 to Setpoint" -> [_ w1202]
          tunnel: "Setpoints (V)" -> [w1190 w1205]
          tunnel: w1179 -> [_ w1199]
          frame False {
            n794 = Multiply(x=3276.7, y=w1190) -> (x*y=w1191:cluster{"Set 1":dbl, "Set 2":dbl})
            n795 = To Word Integer(number=w1191) -> (16bit integer=w1189:cluster{"Set 1":i16, "Set 2":i16})
          }
          frame True {
            n796 = Unbundle By Name(w1199) -> ("Set 1"=w1198:dbl, "Set 2"=w1197:dbl)
            n797 = Unbundle By Name(w1205) -> ("Set 1"=w1204:dbl, "Set 2"=w1203:dbl)
            n798 = Unbundle By Name(w1202) -> ("Set 1"=w1201:bool, "Set 2"=w1200:bool)
            n799 = Select(t=w1198, s=w1201, f=w1204) -> (s? t:f=w1196:dbl)
            n800 = Select(t=w1197, s=w1200, f=w1203) -> (s? t:f=w1195:dbl)
            n801 = Bundle By Name(cluster=w1205, "Set 1"=w1196, "Set 2"=w1195) -> (w1193:cluster{"Set 1":dbl, "Set 2":dbl})
            n802 = local write "Setpoints (V)"(w1193) -> ()
            n803 = Multiply(x=3276.7, y=w1193) -> (x*y=w1194:cluster{"Set 1":dbl, "Set 2":dbl})
            n804 = To Word Integer(number=w1194) -> (16bit integer=w1206:cluster{"Set 1":i16, "Set 2":i16})
          }
        }
        n805 = Unbundle By Name(w1178) -> ("Set 1"=w1177:i16, "Set 2"=w1176:i16)
        n806 = xnode "Read/Write Control"("FPGA VI Reference In"=w1174, "error in"=w1173, "FB Setpoint Set 1"=w1177, "FB Setpoint Set 2"=w1176) -> ("error out"=w1172:errorcluster)  [unwired: 1 out]
      }
      event "Invert GI": Value Change {
        n807 = event-data() -> ()  [unwired: 7 out]
        n808 = xnode "Read/Write Control"("FPGA VI Reference In"=w1211, "error in"=w1209, "Invert GI"="Invert GI", "Invert GI 2"="Invert GI") -> ("error out"=w1210:errorcluster)  [unwired: 1 out]
      }
      event "Green FB Setpoint (mV)", "Green FB Gains", "Green FB On/Off", "Current When FB OFF (%)", "Green int current ON count adj": Value Change {
        n809 = event-data() -> ()  [unwired: 7 out]
        n810 = local read "Green FB Setpoint (mV)"() -> (w1218:dbl)
        n811 = local read "Current When FB OFF (%)"() -> (w1221:dbl)
        n812 = Multiply(x=w1218, y=3.2767) -> (x*y=w1217:dbl)
        n813 = Multiply(x=w1221, y=655.35) -> (x*y=w1222:dbl)
        n814 = To Unsigned Word Integer(number=w1222) -> (unsigned 16bit integer=w1220:u16)
        n815 = local read "Green int current ON count adj"() -> (w1225:u32)
        n816 = local read "Green FB Gains"() -> (w1224:T14)
        n817 = local read "Green Laser ON/Interlacing"() -> (w1215:bool)
        n818 = local read "Green laser mode"() -> (w1214:enum32{"Laser ON", "Laser OFF", "Interlace"})
        n819 = local read "Green FB On/Off"() -> (w1226:bool)
        n820 = Equal?(x=w1214, y=enum32{"Laser ON", "Laser OFF", "Interlace"}."Interlace") -> (x = y?=w1212:bool)
        n821 = Compound Arithmetic op=AND(w1212, w1226, w1215) -> (w1216:bool)
        n822 = xnode "Read/Write Control"("FPGA VI Reference In"=w1229, "error in"=w1228, "Green FB Setpoint"=w1217, "Green FB On/Off"=w1216, "Current Out"=w1220, "Green int current ON count adj"=w1225, "Green FB Gains"=w1224) -> ("error out"=w1227:errorcluster)  [unwired: 1 out]
      }
      event "Green laser mode", "Green Laser ON/Interlacing": Value Change {
        n823 = event-data() -> ()  [unwired: 7 out]
        n824 = case shown="True" "Green Laser ON/Interlacing" {
          tunnel: "Green laser mode" -> [_ w1243]
          tunnel: [enum32{"Laser ON", "Laser OFF", "Interlace"}."Laser OFF" ("Green laser mode") w1243] -> w1231
          tunnel: [FALSE w1239] -> w1230
          frame False {
          }
          frame True {
            n825 = local read "Green FB On/Off"() -> (w1240:bool)
            n826 = Equal?(x=w1243, y=enum32{"Laser ON", "Laser OFF", "Interlace"}."Interlace") -> (x = y?=w1241:bool)
            n827 = And(x=w1241, y=w1240) -> (x .and. y?=w1239:bool)
          }
        }
        n828 = xnode "Read/Write Control"("FPGA VI Reference In"=w1236, "error in"=w1234, "Operating Mode"=w1231, "Operating Mode 2"=w1231, "Green FB On/Off"=w1230) -> ("error out"=w1235:errorcluster)  [unwired: 1 out]
      }
      event "Test ttrig": Value Change {
        n829 = event-data() -> ()  [unwired: 7 out]
        n830 = xnode "Read/Write Control"("FPGA VI Reference In"=w1247, "error in"=w1246, "TTrig?"=TRUE) -> ("error out"=w1245:errorcluster)  [unwired: 1 out]
      }
      event "Neg. TTrig FPGA": Value Change {
        n831 = event-data() -> ()  [unwired: 7 out]
        n832 = xnode "Read/Write Control"("FPGA VI Reference In"=w1251, "error in"=w1250, "TTrig Negate Pos"="Neg. TTrig FPGA") -> ()  [unwired: 2 out]
      }
      event "- phase (APD 1 Gate)", "+ phase (APD 1 Gate)": Value Change {
        n833 = event-data() -> ()  [unwired: 7 out]
        n834 = local read "Phase Adj. (APD 1 Gate)"() -> (w1252:i16)
        n835 = Negate(x=w1252) -> (-x=w1260:i16)
        n836 = Select(t=w1260, s="- phase (APD 1 Gate)", f=w1252) -> (s? t:f=w1259:i16)
        n837 = Or(x="- phase (APD 1 Gate)", y="+ phase (APD 1 Gate)") -> (x .or. y?=w1255:bool)
        n838 = xnode "Read/Write Control"("FPGA VI Reference In"=w1262, "error in"=w1261, "Phase count adjustment (APD 1 Gate)"=w1259) -> ("FPGA VI Reference Out"=w1257:T19, "error out"=w1258:errorcluster)
        n839 = xnode "Read/Write Control"("FPGA VI Reference In"=w1257, "error in"=w1258, "+ phase (APD 1 Gate)"=w1255) -> ("error out"=w1256:errorcluster)  [unwired: 1 out]
      }
      event "+ phase (APD 2 Gate)", "- phase (APD 2 Gate)": Value Change {
        n840 = event-data() -> ()  [unwired: 7 out]
        n841 = local read "Phase Adj. (APD 2 Gate)"() -> (w1263:i16)
        n842 = Negate(x=w1263) -> (-x=w1271:i16)
        n843 = Select(t=w1271, s="- phase (APD 2 Gate)", f=w1263) -> (s? t:f=w1270:i16)
        n844 = Or(x="- phase (APD 2 Gate)", y="+ phase (APD 2 Gate)") -> (x .or. y?=w1266:bool)
        n845 = xnode "Read/Write Control"("FPGA VI Reference In"=w1273, "error in"=w1272, "Phase count adjustment (APD 2 Gate)"=w1270) -> ("FPGA VI Reference Out"=w1268:T19, "error out"=w1269:errorcluster)
        n846 = xnode "Read/Write Control"("FPGA VI Reference In"=w1268, "error in"=w1269, "+ phase (APD 2 Gate)"=w1266) -> ("error out"=w1267:errorcluster)  [unwired: 1 out]
      }
      event "Phase Adj. (APD Acq)", "+ phase (APD Acq)", "- phase (APD Acq)": Value Change {
        n847 = event-data() -> ()  [unwired: 7 out]
        n848 = local read "Phase Adj. (APD Acq)"() -> (w1276:i16)
        n849 = Negate(x=w1276) -> (-x=w1282:i16)
        n850 = Select(t=w1282, s="+ phase (APD Acq)", f=w1276) -> (s? t:f=w1281:i16)
        n851 = Or(x="+ phase (APD Acq)", y="- phase (APD Acq)") -> (x .or. y?=w1277:bool)
        n852 = xnode "Read/Write Control"("FPGA VI Reference In"=w1284, "error in"=w1283, "Phase Count Adjustment (APD Acq)"=w1281) -> ("FPGA VI Reference Out"=w1279:T19, "error out"=w1280:errorcluster)
        n853 = xnode "Read/Write Control"("FPGA VI Reference In"=w1279, "error in"=w1280, "+ phase (APD Acq)"=w1277) -> ("error out"=w1278:errorcluster)  [unwired: 1 out]
      }
      event "Phase adj. (GI)", "+ phase (GI)", "- phase (GI)": Value Change {
        n854 = event-data() -> ()  [unwired: 7 out]
        n855 = Negate(x="Phase adj. (GI)") -> (-x=w1293:i16)
        n856 = Select(t=w1293, s="+ phase (GI)", f="Phase adj. (GI)") -> (s? t:f=w1292:i16)
        n857 = Or(x="+ phase (GI)", y="- phase (GI)") -> (x .or. y?=w1288:bool)
        n858 = xnode "Read/Write Control"("FPGA VI Reference In"=w1295, "error in"=w1294, "Phase count adjustment (GI)"=w1292) -> ("FPGA VI Reference Out"=w1290:T19, "error out"=w1291:errorcluster)
        n859 = xnode "Read/Write Control"("FPGA VI Reference In"=w1290, "error in"=w1291, "+ phase (GI)"=w1288) -> ("error out"=w1289:errorcluster)  [unwired: 1 out]
      }
      event "Phase adj. (GI) 2", "+ phase (GI) 2", "- phase (GI) 2": Value Change {
        n860 = event-data() -> ()  [unwired: 7 out]
        n861 = Negate(x="Phase adj. (GI) 2") -> (-x=w1304:i16)
        n862 = Select(t=w1304, s="+ phase (GI) 2", f="Phase adj. (GI) 2") -> (s? t:f=w1303:i16)
        n863 = Or(x="+ phase (GI) 2", y="- phase (GI) 2") -> (x .or. y?=w1299:bool)
        n864 = xnode "Read/Write Control"("FPGA VI Reference In"=w1306, "error in"=w1305, "Phase count adjustment (GI) 2"=w1303) -> ("FPGA VI Reference Out"=w1301:T19, "error out"=w1302:errorcluster)
        n865 = xnode "Read/Write Control"("FPGA VI Reference In"=w1301, "error in"=w1302, "+ phase (GI) 2"=w1299) -> ("error out"=w1300:errorcluster)  [unwired: 1 out]
      }
      event "Phase adj. (Green FB)", "- phase (Green FB)", "+ phase (Green FB)": Value Change {
        n866 = event-data() -> ()  [unwired: 7 out]
        n867 = Negate(x="Phase adj. (Green FB)") -> (-x=w1315:i16)
        n868 = Select(t=w1315, s="+ phase (Green FB)", f="Phase adj. (Green FB)") -> (s? t:f=w1314:i16)
        n869 = Or(x="+ phase (Green FB)", y="- phase (Green FB)") -> (x .or. y?=w1310:bool)
        n870 = xnode "Read/Write Control"("FPGA VI Reference In"=w1317, "error in"=w1316, "Phase count adjustment (Green FB)"=w1314) -> ("FPGA VI Reference Out"=w1312:T19, "error out"=w1313:errorcluster)
        n871 = xnode "Read/Write Control"("FPGA VI Reference In"=w1312, "error in"=w1313, "+ phase (Green FB)"=w1310) -> ("error out"=w1311:errorcluster)  [unwired: 1 out]
      }
      event "Invert APD Gate", "APD Gate ON Count", "APD Gate OFF Count", "APD Gate", "APD Integration Time (s)", "APD 1 AO Mult.", "APD 2 AO Mult.", "On one out of X cycles": Value Change {
        n872 = event-data() -> ()  [unwired: 7 out]
        n873 = Add(x="GI Frequency, ON count", y="GI Frequency, OFF count") -> (x+y=w1321:u32)
        n874 = Add(x="APD Gate ON Count", y="APD Gate OFF Count") -> (x+y=w1334:u32)
        n875 = Multiply(x="On one out of X cycles", y=w1321) -> (x*y=w1318:u32)
        "Green FB Count" <- w1318
        n876 = Subtract(x=w1318, y="GI Frequency, ON count") -> (x-y=w1319:u32)
        n877 = Multiply(x=w1334, y="On one out of X cycles") -> (x*y=w1333:u32)
        n878 = Subtract(x=w1333, y="APD Gate ON Count") -> (x-y=w1332:u32)
        n879 = local read "DMA Update Period (s)"() -> (w1335:dbl)
        n880 = Multiply(x="APD Integration Time (s)", y=40000000.0) -> (x*y=w1340:dbl)
        n881 = Reciprocal(x="APD Integration Time (s)") -> (1/x=→"APD Acq Rate (Hz)":dbl)
        n882 = To Unsigned Long Integer(number=w1340) -> (unsigned 32bit integer=w1324:u32)
        "APD Int. Count" <- w1324
        n883 = xnode "Read/Write Control"("FPGA VI Reference In"=w1344, "error in"=w1343, "Invert APD Gate"="Invert APD Gate", "APD Gate ON Count"="APD Gate ON Count", "APD Gate OFF Count"=w1332, "APD Acq Rate Count"=w1324, "APD Gate Operating Mode"="APD Gate", "APD 1 AO scale factor"="APD 1 AO Mult.", "APD 2 AO scale factor"="APD 2 AO Mult.", "Green interlace ON count"="GI Frequency, ON count", "Green interlace OFF count"=w1319, "Green interlace ON count 2"="GI Frequency, ON count", "Green interlace OFF count 2"=w1319, "Green FB Count"=w1318) -> ("error out"=w1342:errorcluster)  [unwired: 1 out]
        n884 = Divide(x=w1335, y="APD Integration Time (s)") -> (x/y=w1338:dbl)
        n885 = Multiply(x=2.0, y=w1338) -> (x*y=w1337:dbl)
        n886 = local write "APD Samples/FIFO Acq."(w1338) -> ()
        n887 = local write "APD Elements/DMA read"(w1337) -> ()
      }
      event "Number of F/B Scans (AOD)", "Scan Speed (nm/s)", "Scan BD", "Initial delta (MHz)", "Step Size (nm)", "Scan Range (nm)": Value Change {
        w1406 = 123.0  # AOM cal (nm/MHz)
        n888 = event-data() -> ()  [unwired: 7 out]
        n889 = local read "BD 1 Frequency 1 (MHz)"() -> (w1389:dbl)
        n890 = local read "AOM X Cal (nm/MHz)"() -> (w1381:dbl)
        n891 = local read "X RF Frequency Limits (MHz)"() -> (w1393:T16)
        n892 = local read "Y RF Frequency Limits (MHz)"() -> (w1390:T16)
        n893 = local read "BD 2 Frequency 1 (MHz)"() -> (w1395:dbl)
        n894 = Negate(x="Scan Range (nm)") -> (-x=w1359:dbl)
        n895 = Divide(x=w1359, y=w1381) -> (x/y=w1363:dbl)
        n896 = Select(t=w1393, s="Scan BD", f=w1390) -> (s? t:f=w1392:T16)
        n897 = Select(t=w1389, s="Scan BD", f=w1395) -> (s? t:f=w1394:dbl)
        n898 = Unbundle By Name(w1392) -> ("Maximum"=w1401:dbl, "Minimum"=w1400:dbl)
        n899 = Add(x=w1363, y=w1394) -> (x+y=w1398:dbl)
        n900 = Divide(x=w1359, y="Step Size (nm)") -> (x/y=w1378:dbl)
        n901 = Divide(x="Step Size (nm)", y=w1381) -> (x/y=w1387:dbl)
        n902 = Absolute Value(x=w1378) -> (abs(x)=w1362:dbl)
        n903 = Sign(1:w1359) -> (0:w1360:dbl)
        n904 = In Range and Coerce(upper limit=w1401, x=w1398, lower limit=w1400) -> (coerced(x)=w1397:dbl, In Range?=w1399:bool)
        n905 = To Unsigned Quad Integer(1:w1362) -> (0:w1377:u64)
        "Scan steps (AOD)" <- w1377
        n906 = call "IR AOM freq to word.vi"("Frequency In (MHz)"=w1387) -> ("Frequency Word Out (double)"=w1384:dbl)
        n907 = Multiply(x=w1360, y=w1384) -> (x*y=w1361:dbl)
        n908 = Subtract(x=w1398, y=w1397) -> (x-y=w1396:dbl)
        n909 = To Quad Integer(1:w1361) -> (0:w1383:i64)
        "Incr. int (AOD)" <- w1383
        n910 = Subtract(x=w1363, y=w1396) -> (x-y=w1382:dbl)
        "Scan Range (MHz)" <- w1382
        n911 = Select(t=w1363, s=w1399, f=w1382) -> (s? t:f=w1402:dbl)
        n912 = Multiply(x=w1382, y=w1381) -> (x*y=w1380:dbl)
        n913 = Decrement(x=w1377) -> (x-1=w1430:u64)
        n914 = Negate(x=w1380) -> (-x=w1376:dbl)
        n915 = local write "Scan Range (nm)"(w1376) -> ()
        n916 = Divide(x=w1402, y=w1430) -> (x/y=w1386:dbl)
        "Scan Increment (MHz)" <- w1386
        n917 = call "IR AOM freq to word.vi"("Frequency In (MHz)"=w1386) -> ("Frequency Word Out (double)"=w1385:dbl)
        n918 = Divide(x="Step Size (nm)", y="Scan Speed (nm/s)") -> (x/y=w1373:dbl)
        n919 = To Quad Integer(1:w1385) -> ()  [unwired: 1 out]
        n920 = local read "Number Interlace Sets"() -> (w1357:u8)
        n921 = local read "AI Count (ticks)"() -> (w1358:u32)
        n922 = local read "Total Counts (ticks)"() -> (w1356:u32)
        n923 = local read "# Samples/trap"() -> (w1388:u32)
        n924 = Multiply(x=w1358, y=w1357) -> (x*y=w1355:u32)
        n925 = Divide(x=w1356, y=w1355) -> (x/y=w1354:dbl)
        n926 = Select(t=w1389, s="Scan BD", f=w1395) -> (s? t:f=w1427:dbl)
        "Initial freq. (MHz)" <- w1427
        n927 = Add(x=w1402, y=w1427) -> (x+y=→"Final freq. (MHz)":dbl)
        n928 = Divide(x=w1356, y=40000000.0) -> (x/y=w1372:dbl)
        n929 = Divide(x=w1373, y=w1372) -> (x/y=w1371:dbl)
        n930 = To Unsigned Quad Integer(1:w1371) -> (0:w1346:u64)
        n931 = Quotient & Remainder(x=w1346, y=u64 2) -> (x-y*floor(x/y)=w1350:u64)  [unwired: 1 out]
        n932 = Equal?(x=w1350, y=u64 0) -> (x = y?=w1348:bool)
        n933 = Decrement(x=w1346) -> (x-1=w1347:u64)
        n934 = Select(t=w1346, s=w1348, f=w1347) -> (s? t:f=w1345:u64)
        "Cycles/step (AOD)" <- w1345
